vi "cm_Channel Monitor Uninit.vi"(2 "Container State":T1, 3 "Display State":T2={"Chan"=[], "First Drop?"=FALSE, "Notifier Name"="", "Refresh View"=FALSE, "Scale to Input Range"=FALSE, "Linear View"=FALSE, "Display"={"Current"=6618880, "Peak"=6618880}, "Property/Method"=enum."No Update", "Time Display Ref"=[]}) -> ()   [LabVIEW 2012, in "Channel Monitor.xctl"]
uses:
  Channel Monitor.xctl
  cm_Channel Monitor State.ctl
  TypeDef/cm_Property_Method.ctl
  <vilib>/_xctls/Container State.ctl
  cm_XControlState Action.ctl
  <vilib>/_xctls/XControlSupport.lvlib
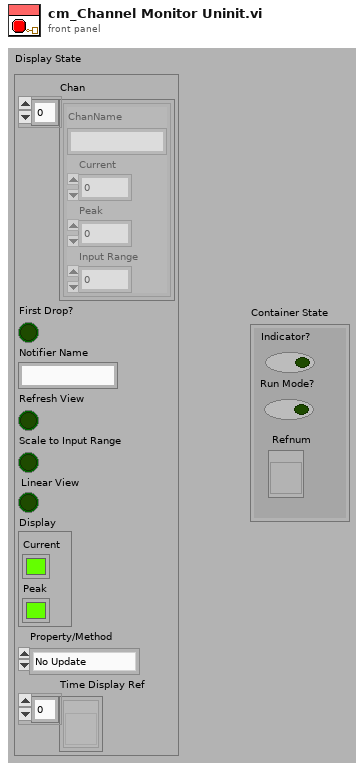
[diagram p1: front panel]
types:
  T1 = typedef "XControlSupport.lvlib/Container State.ctl" = cluster{"Indicator?":bool, "Run Mode?":bool, " Refnum":refnum<vi>}
  T2 = typedef "Channel Monitor.xctl/cm_Channel Monitor State.ctl" = cluster{"Chan":cluster{"ChanName":string, "Current":dbl, "Peak":dbl, "Input Range":dbl}[], "First Drop?":bool, "Notifier Name":string, "Refresh View":bool, "Scale to Input Range":bool, "Linear View":bool, "Display":cluster{"Current":u32, "Peak":u32}, "Property/Method":T3, "Time Display Ref":refnum<vi>[]}
  T3 = typedef "Channel Monitor.xctl/cm_Property_Method.ctl" = enum16{"No Update", "Color: Currrent", "Color: Peak", "Close Time Displays"}
  T4 = typedef "Channel Monitor.xctl/cm_XControlState Action.ctl" = enum16{"Add", "Write", "Read", "Remove"}
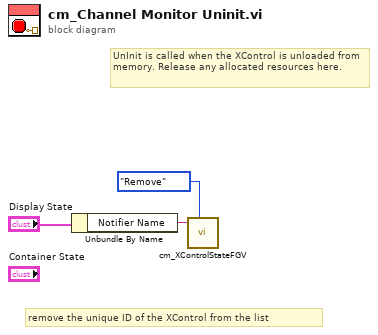
[diagram p0: block diagram]
diagram:
  # "remove the unique ID of the XControl from the list"
  # "UnInit is called when the XControl is unloaded from memory. Release any allocated resources here."
  n1 = Unbundle By Name("Display State") -> ("Notifier Name"=w1:string)
  n2 = call "cm_XControlStateFGV.vi"("Action"=cm_XControlState_Action."Remove", "XControl Name"=w1) -> ()  [unwired: 6 in, 4 out]
